vi "Testing.vi"() -> ()   [LabVIEW 2020]
uses:
  Msg Set.ctl
  Msg/Msg.lvclass
  Actor.lvlib
panel:
  out "Array 2":path[](array[path])
  out "Array":string[](array[string])
  out "Local Msg Set":T1
  out "parent interfaces":variant[](array[variant])
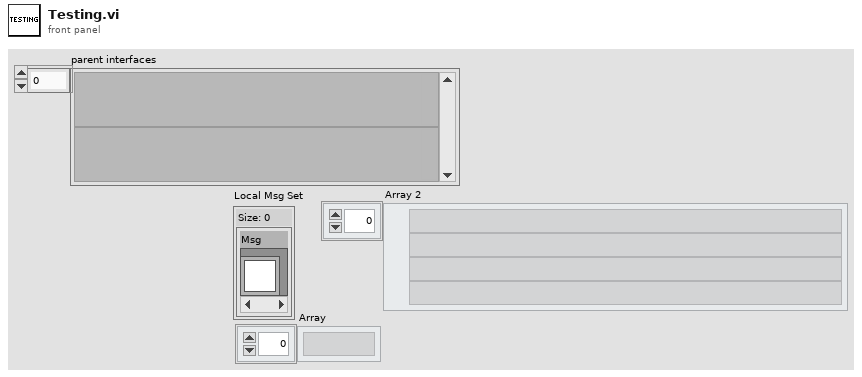
[diagram p1: front panel]
types:
  T1 = typedef "jettl.lvlib/Actor.lvlib/Msg Set.ctl" = set{refnum<class "Msg.lvclass">}
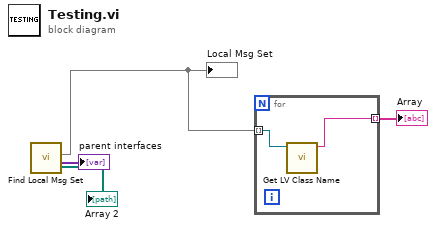
[diagram p0: block diagram]
diagram:
  n1 = call "Find Local Msg Set.vi"() -> ("parent interfaces"=→"parent interfaces":variant[], "Local Msg Set"=w3:T1, "Array"=→"Array 2":path[], "Variant (Actor)"=w5:variant)  [unwired: 7 in, 1 out]
  "Local Msg Set" <- w3
  n2 = for {
    tunnel: w3 -> [w7] mode=indexing
    tunnel: [w6] -> w2 mode=indexing
    n3 = call <vilib>:"Get LV Class Name.vi"("object"=w7) -> ("class name"=w6:string)  [unwired: 9 in, 1 out]
  }
  "Array" <- w2
